vi "Delay over UDP(Tx).vi"(3 "local port(Rx)":u16=54323, 4 "remote port":u16=54322, 5 "remote IP Address":string="192.168.10.3", 6 "Iteration":i32=100) -> (0 "Array 2":cluster{"ID":string, "Timestamp":u32}[](array[cluster]), 1 "Array":cluster{"ID":string, "Timestamp":u32}[](array[cluster]), 2 "Output":i32[](array[numeric]))   [LabVIEW 2014]
panel:
  out "Mean":dbl
  out "error out(RX)":errorcluster
  out "error out(TX)":errorcluster
  in  "local port(Tx)":u16=54321
  out "possibility":i32
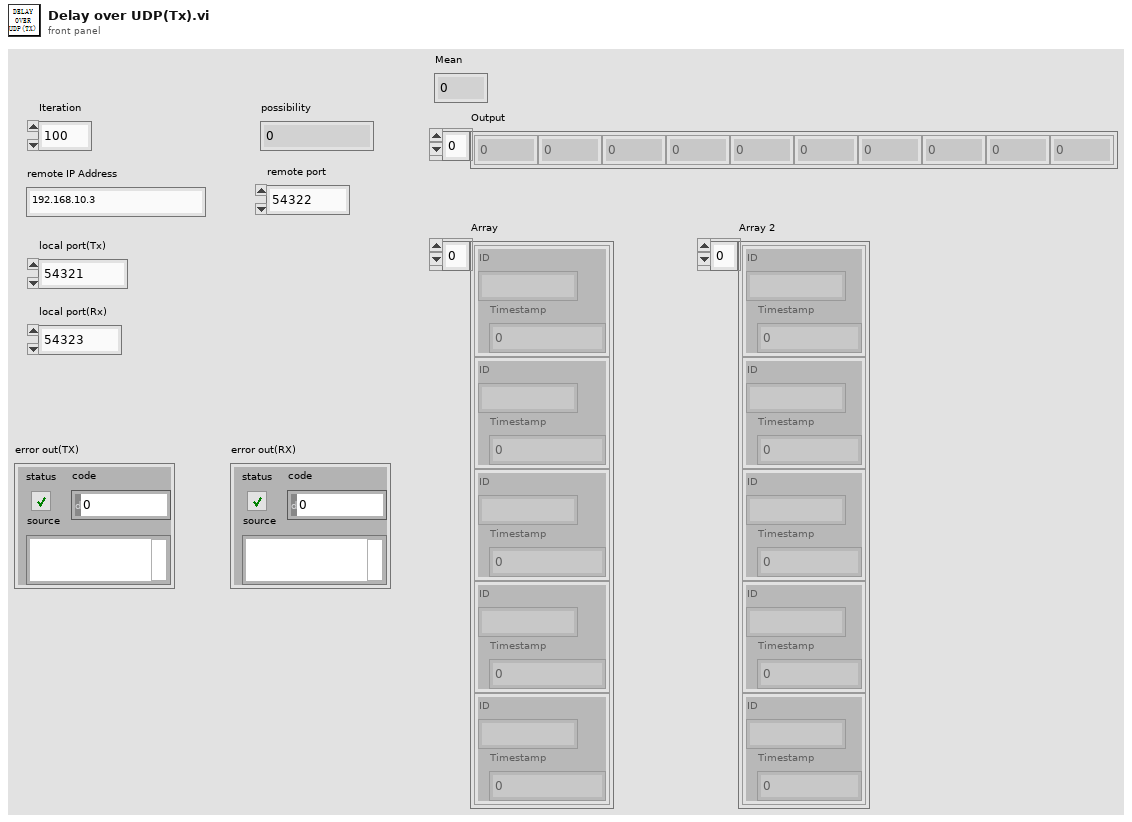
[diagram p1: front panel]
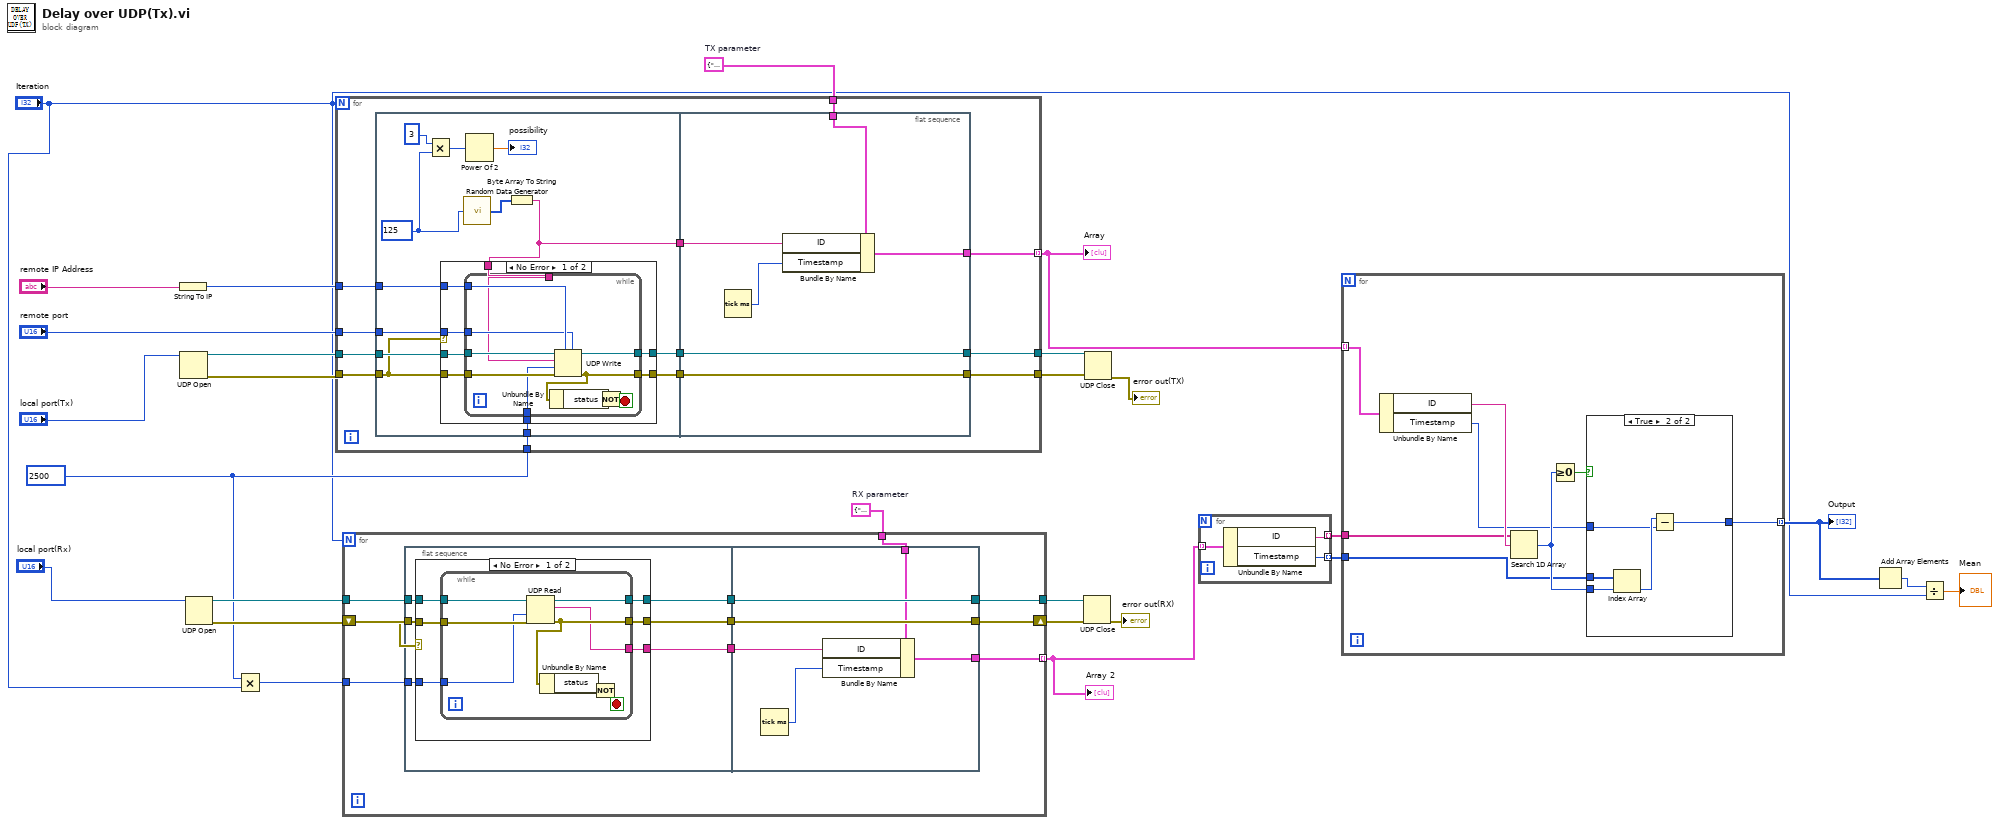
[diagram p0: block diagram]
diagram:
  w6 = 2500 ("timeout ms (25000)")
  w13 = cluster{"ID":string, "Timestamp":u32} {"ID"="string", "Timestamp"=0}  # RX parameter
  w18 = cluster{"ID":string, "Timestamp":u32} {"ID"="string", "Timestamp"=0}  # TX parameter
  n1 = String To IP(1:"remote IP Address") -> (0:w25:u32)
  n2 = UDP Open(11:"local port(Tx)") -> (port=w22:refnum<k16>, 0:w27:errorcluster)  [unwired: 4 in, 1 out]
  n3 = UDP Open(11:"local port(Rx)") -> (port=w17:refnum<k16>, 0:w16:errorcluster)  [unwired: 4 in, 1 out]
  n4 = Multiply(x=w6, y="Iteration") -> (x*y=w5:i32)
  n5 = for {
    N: "Iteration" -> [_]
    tunnel: w25 -> [w38]
    tunnel: "remote port" -> [w37]
    tunnel: w22 -> [w36]
    tunnel: [w35] -> w20
    tunnel: w18 -> [w31]
    tunnel: [w29] -> w12 mode=indexing
    tunnel: w27 -> [w39]
    tunnel: [w34] -> w21
    tunnel: w6 -> [w28]
    n6 = flat-sequence {
      tunnel: w39 -> [w41]
      tunnel: w38 -> [w48]
      tunnel: w37 -> [w47]
      tunnel: w36 -> [w46]
      tunnel: [w44] -> w33
      tunnel: [w43] -> w32
      tunnel: [w42] -> w30
      tunnel: w28 -> [w40]
      tunnel: [w74] -> w34
      tunnel: [w78] -> w35
      tunnel: w33 -> [w78]
      tunnel: w32 -> [w74]
      tunnel: w31 -> [w77]
      tunnel: w30 -> [w76]
      tunnel: [w75] -> w29
      frame #0 {
        w45 = 125 ("number of samples")
        n7 = Multiply(x=3, y=w45) -> (x*y=w51:i32)
        n8 = call "Random Data Generator.vi"("Data Length"=w45) -> ("Data"=w49:u8[])
        n9 = Power Of 2(x=w51) -> (2^x=→"possibility":dbl)
        n10 = Byte Array To String(unsigned byte array=w49) -> (string=w42:string)
        n11 = case shown="No Error" w41 {
          tunnel: w41 -> [w60 w72]
          tunnel: w48 -> [w59 _]
          tunnel: w47 -> [w58 _]
          tunnel: w46 -> [w57 w71]
          tunnel: [w56 w71] -> w44
          tunnel: [w55 w72] -> w43
          tunnel: w42 -> [w54 _]
          tunnel: w40 -> [w53 _]
          frame No Error {
            n12 = while {
              tunnel: w59 -> [w69]
              tunnel: w58 -> [w68]
              tunnel: w54 -> [w65]
              tunnel: w57 -> [w67]
              tunnel: [w66] -> w56
              tunnel: w60 -> [w70]
              tunnel: [w64] -> w55
              tunnel: w53 -> [w61]
              stop <- w62 stop-if-true
              n13 = UDP Write(address=w69, port or service name=w68, connection ID=w67, data in=w65, 8:w70, 9:w61) -> (error out=w64:errorcluster, 3:w66:refnum<k16>)
              n14 = Unbundle By Name(w64) -> ("status"=w63:bool)
              n15 = Not(x=w63) -> (.not. x?=w62:bool)
            }
          }
          frame Error {
          }
        }
      }
      frame #1 {
        n16 = Tick Count (ms)() -> (millisecond timer value=w73:u32)
        n17 = Bundle By Name(cluster=w77, "ID"=w76, "Timestamp"=w73) -> (w75:cluster{"ID":string, "Timestamp":u32})
      }
    }
  }
  "Array" <- w12
  n18 = for {
    N: "Iteration" -> [_]
    tunnel: w17 -> [w88]
    tunnel: [w87] -> w15
    shift-right: [w86] -> w14
    shift-left: w16 -> [w85]
    tunnel: w13 -> [w82]
    tunnel: [w80] -> w11 mode=indexing
    tunnel: w5 -> [w79]
    n19 = flat-sequence {
      tunnel: w88 -> [w94]
      tunnel: w85 -> [w91]
      tunnel: [w93] -> w84
      tunnel: [w92] -> w83
      tunnel: [w90] -> w81
      tunnel: w79 -> [w89]
      tunnel: [w115] -> w86
      tunnel: [w116] -> w87
      tunnel: w84 -> [w116]
      tunnel: w83 -> [w115]
      tunnel: w82 -> [w114]
      tunnel: w81 -> [w113]
      tunnel: [w111] -> w80
      frame #0 {
        n20 = case shown="No Error" w91 {
          tunnel: w94 -> [w100 w109]
          tunnel: w91 -> [w99 w110]
          tunnel: [w98 w109] -> w93
          tunnel: [w97 w110] -> w92
          tunnel: [w96 _] -> w90
          tunnel: w89 -> [w95 _]
          frame No Error {
            n21 = while {
              tunnel: w99 -> [w107]
              tunnel: w100 -> [w108]
              tunnel: [w106] -> w98
              tunnel: [w105] -> w97
              tunnel: [w103] -> w96
              tunnel: w95 -> [w101]
              stop <- w102 stop-if-true
              n22 = UDP Read(connection ID=w108, timeout ms (25000)=w101, 8:w107) -> (data out=w103:string, error out=w105:errorcluster, 3:w106:refnum<k16>)  [unwired: 1 in, 2 out]
              n23 = Unbundle By Name(w105) -> ("status"=w104:bool)
              n24 = Not(x=w104) -> (.not. x?=w102:bool)
            }
          }
          frame Error {
          }
        }
      }
      frame #1 {
        n25 = Tick Count (ms)() -> (millisecond timer value=w112:u32)
        n26 = Bundle By Name(cluster=w114, "ID"=w113, "Timestamp"=w112) -> (w111:cluster{"ID":string, "Timestamp":u32})
      }
    }
  }
  "Array 2" <- w11
  n27 = UDP Close(connection ID=w15, 8:w14) -> (error out=→"error out(RX)":errorcluster)  [unwired: 1 out]
  n28 = UDP Close(connection ID=w20, 8:w21) -> (error out=→"error out(TX)":errorcluster)  [unwired: 1 out]
  n29 = for {
    tunnel: w11 -> [w119] mode=indexing
    tunnel: [w118] -> w10 mode=indexing
    tunnel: [w117] -> w9 mode=indexing
    n30 = Unbundle By Name(w119) -> ("ID"=w118:string, "Timestamp"=w117:u32)
  }
  n31 = for {
    tunnel: w12 -> [w127] mode=indexing
    tunnel: w10 -> [w125]
    tunnel: w9 -> [w122]
    tunnel: [w120] -> w4 mode=indexing
    n32 = Unbundle By Name(w127) -> ("ID"=w126:string, "Timestamp"=w121:u32)
    n33 = Search 1D Array(1D array=w125, element=w126) -> (index of element=w123:i32)  [unwired: 1 in]
    n34 = Greater Or Equal To 0?(x=w123) -> (x >= 0?=w124:bool)
    n35 = case shown="True" w124 {
      tunnel: w123 -> [_ w132]
      tunnel: w122 -> [_ w131]
      tunnel: w121 -> [_ w129]
      tunnel: [_ w128] -> w120
      frame False {
      }
      frame True {
        n36 = Index Array(array=w131, index=w132) -> (element=w130:u32)
        n37 = Subtract(x=w130, y=w129) -> (x-y=w128:u32)
      }
    }
  }
  "Output" <- w4
  n38 = Add Array Elements(numeric array=w4) -> (sum=w2:u32)
  n39 = Divide(x=w2, y="Iteration") -> (x/y=→"Mean":dbl)
